vi "RFSG Arbitrary Waveform Generation.vi"(4 "Single Acquisition?":bool, 6 "Power Level (dBm)":dbl=-20.0 format="%_3f", 7 "Selected Waveform":u16(ring) items=["DoubleSideBand", "LowerSideBand", "UpperSideBand"], 8 "error in":errorcluster {"code" format="%.0x"}, 9 "IQ Rate (S/s)":dbl=1000000.0 format="%#.4p", 10 "Center Frequency (Hz)":dbl=1000000000.0 format="%#.4p", 11 "Resource Name":refnum<k15>="RFSG") -> (0 "Error Out":errorcluster, 2 "Actual IQ Rate (S/s)":dbl format="%#.4p", 3 "Frequency Offset":dbl format="%#.4p")   [LabVIEW 2021]
doc: "Demonstrates how to generate an arbitrary waveform. The example lets you choose one of three waveforms to create and write:\n\n + Double Side Band --> two tones around the center frequency.\n + Lower Side Band --> one tone to the left of the center frequency.\n + Upper Side Band --> one tone to the right of the center frequency.\n\nEach waveform is 100 samples long. The waveforms are generated at a frequency of IQ Rate / 100 samples. For a selection of a 100 MS/s IQ Rate, a spectrum analyzer show tones 1 MHz from the specified center frequency."
uses:
  <vilib>/Utility/error.llb/DialogType.ctl
panel:
  in  "Stop":bool
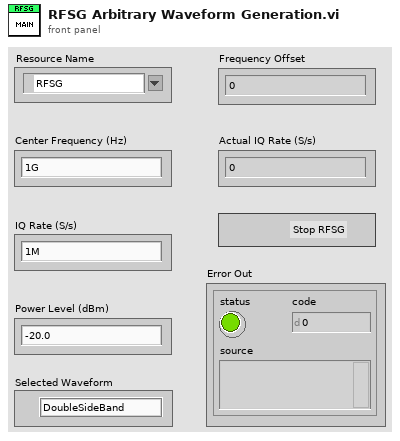
[diagram p1: front panel]
types:
  T1 = typedef "DialogType.ctl" = u16
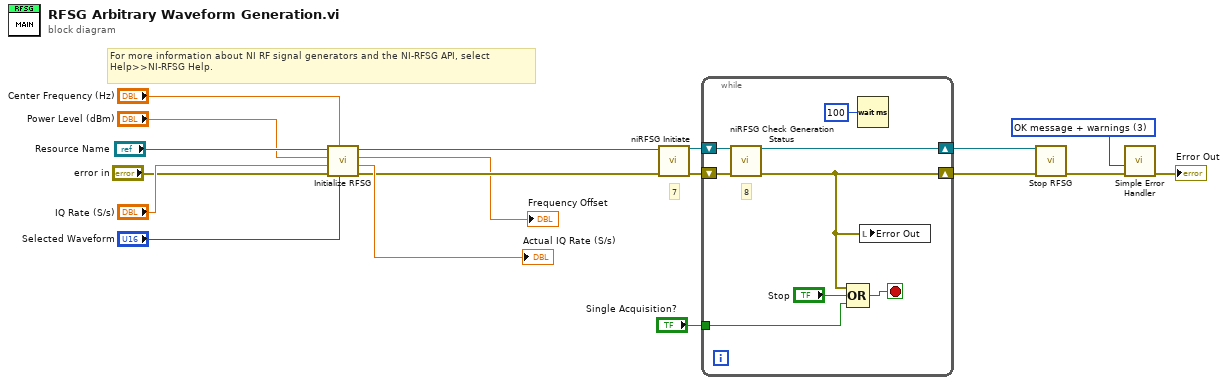
[diagram p0: block diagram]
diagram:
  w5 = T1 3 items=["no dialog", "OK message", "continue or stop message", "OK message + warnings", "continue/stop + warnings"] ("type of dialog (OK msg:1)")
  # "For more information about NI RF signal generators and the NI-RFSG API, select Help>>NI-RFSG Help."
  # "7"
  n1 = call "Initialize RFSG.vi"("Selected Waveform"="Selected Waveform", "Center Frequency"="Center Frequency (Hz)", "error in (no error)"="error in", "IQ Rate"="IQ Rate (S/s)", "Power Level"="Power Level (dBm)", "RFSG Reference In"="Resource Name") -> ("error out"=w13:errorcluster, "Actual IQ Rate (S/s)"=→"Actual IQ Rate (S/s)":dbl, "Frequecy Offset"=→"Frequency Offset":dbl, "RFSG Reference Out"=w14:refnum<k15>)  [unwired: 2 in]
  n2 = call <instrlib>:"niRFSG Initiate.vi"("instrument handle"=w14, "error in"=w13) -> ("instrument handle out"=w18:refnum<k15>, "error out"=w6:errorcluster)  [unwired: 12 in]
  n3 = while {
    shift-right: [w22] -> w17
    shift-left: w18 -> [w23]
    shift-right: [w20] -> w7
    shift-left: w6 -> [w21]
    tunnel: "Single Acquisition?" -> [w19]
    stop <- w25 stop-if-true
    # "8"
    n4 = call <instrlib>:"niRFSG Check Generation Status.vi"("instrument handle"=w23, "error in"=w21) -> ("instrument handle out"=w22:refnum<k15>, "error out"=w20:errorcluster)  [unwired: 11 in, 1 out]
    n5 = Compound Arithmetic op=OR(w20, "Stop", w19) -> (w25:bool)
    n6 = Wait (ms)(milliseconds to wait=u32 100) -> ()  [unwired: 1 out]
    n7 = local write "Error Out"(w20) -> ()
  }
  n8 = call "Stop RFSG.vi"("error in (no error)"=w7, "RFSG Reference In"=w17) -> ("error out"=w4:errorcluster)  [unwired: 9 in]
  n9 = call <vilib>:"Simple Error Handler.vi"("type of dialog (OK msg:1)"=w5, "error in (no error)"=w4) -> ("error out"=→"Error Out":errorcluster)  [unwired: 3 in, 4 out]
